vi "Check_Motility_after_Gap_Closing-2.vi"(0 "(X,Y) IN":dbl[][](array[numeric]), 1 "dR min":dbl, 5 "??? Gap closed potentially ???":bool, 7 "X":dbl, 9 "Y":dbl, 11 "Count of \ngaps between\ndots":i32, 12 "i+j (index\nof dot before\ngap closing)":i32) -> (4 "Gap closed!!!":bool, 6 "X OUT":dbl, 8 "Y OUT":dbl, 10 "[OUT] Count \nof gapes + \nnext dot in \nsearching":i32, 14 "[OUT] current dot\n# frame (column)":i32, 15 "[OUT] current # dot\nin the frame (column)":i32)   [LabVIEW 2013]
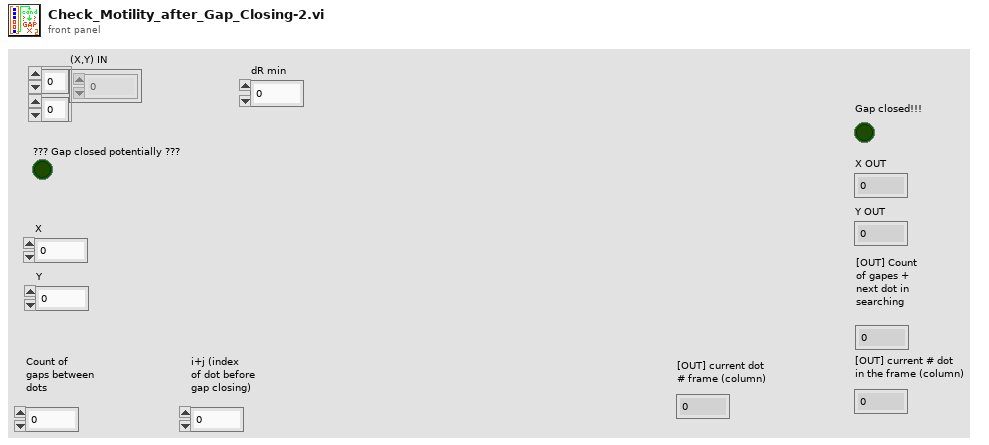
[diagram p1: front panel]
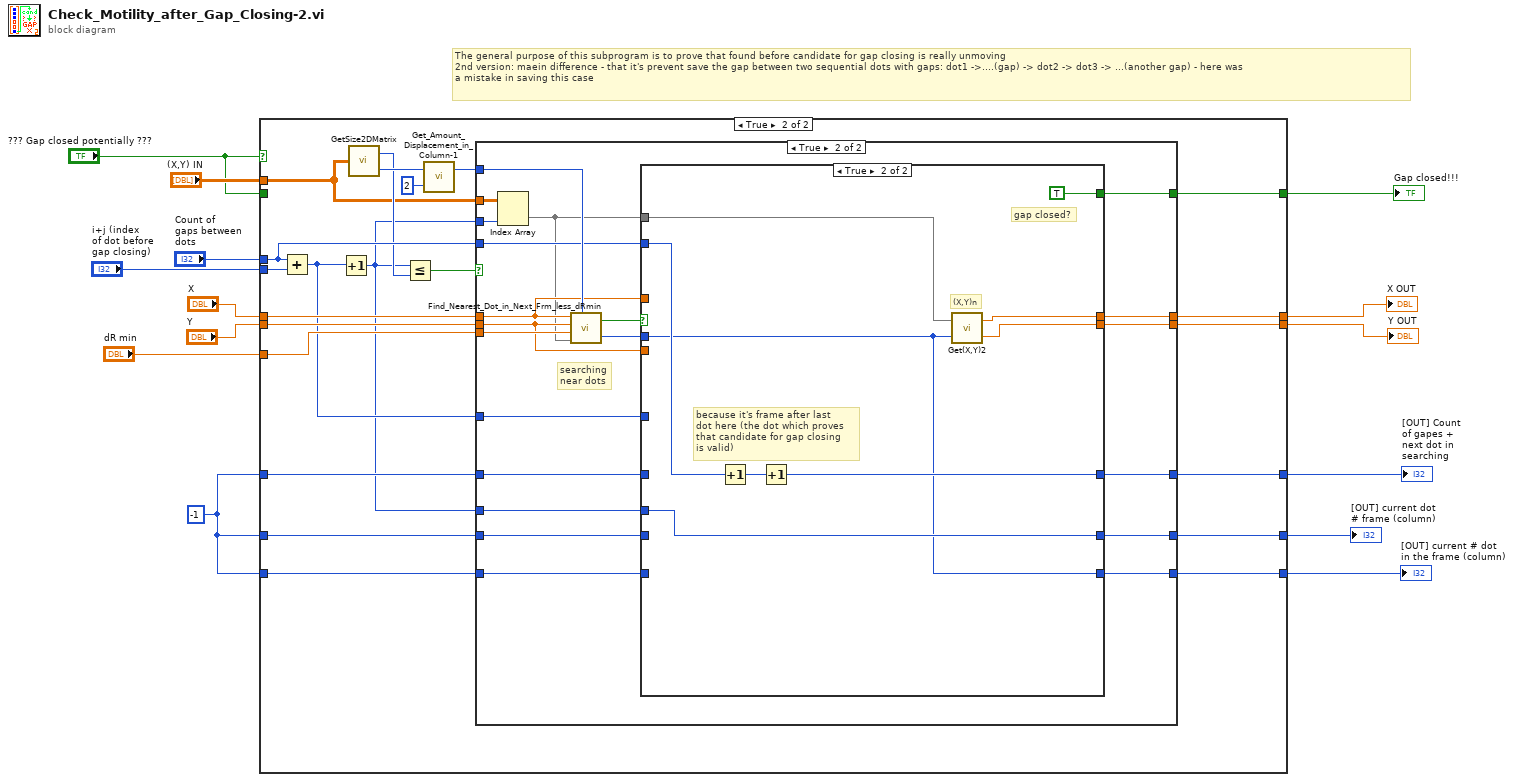
[diagram p0: block diagram]
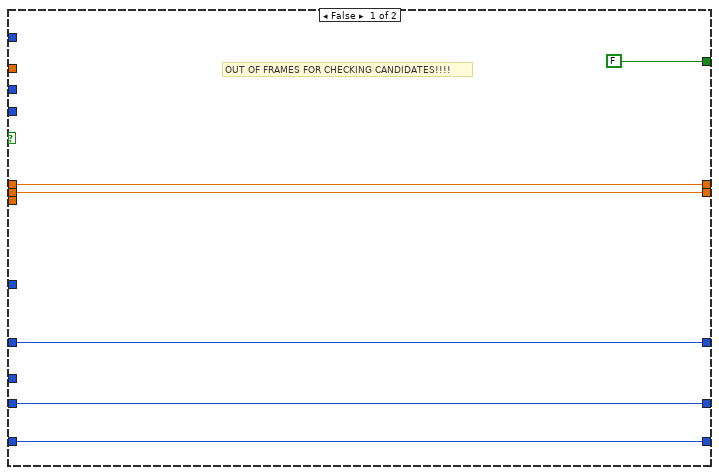
[diagram p3: hidden frame]
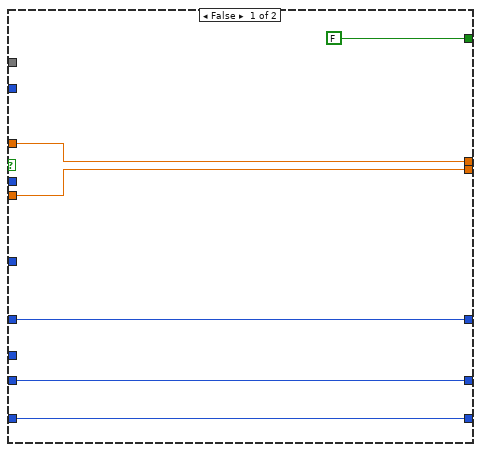
[diagram p4: hidden frame]
diagram:
  w1 = -1
  # "The general purpose of this subprogram is to prove that found before candidate for gap closing is really unmoving\n2nd version: maein difference - that it's prevent save the gap between two sequential dots with gaps: dot1 ->....(gap) -> dot2 -> dot3 -> ...(another gap) - here was\na mistake in saving this case"
  n1 = case shown="True" "??? Gap closed potentially ???" {
    tunnel: "X" -> [w20 w36]
    tunnel: "Y" -> [w19 w35]
    tunnel: "(X,Y) IN" -> [_ w22]
    tunnel: "i+j (index\nof dot before\ngap closing)" -> [_ w42]
    tunnel: "Count of \ngaps between\ndots" -> [_ w37]
    tunnel: "dR min" -> [_ w38]
    tunnel: [w20 w32] -> w8
    tunnel: [w19 w31] -> w7
    tunnel: "??? Gap closed potentially ???" -> [w18 _]
    tunnel: [w18 w33] -> w5
    tunnel: w1 -> [w17 w30]
    tunnel: [w17 w29] -> w4
    tunnel: w1 -> [w16 w28]
    tunnel: w1 -> [w15 w27]
    tunnel: [w16 w26] -> w3
    tunnel: [w15 w25] -> w2
    frame False {
    }
    frame True {
      n2 = Add(x=w37, y=w42) -> (x+y=w34:i32)
      n3 = Increment(x=w34) -> (x+1=w21:i32)
      n4 = call "GetSize2DMatrix.vi"("Array IN (2D)"=w22) -> ("# Cols"=w23:i32, "# Rows"=w41:i32)
      n5 = Less Or Equal?(x=w21, y=w23) -> (x <= y?=w24:bool)
      n6 = call "Get_Amount_Displacement_in_Column-1.vi"("multiplier"=2 ("y"), "# Rows"=w41) -> ("Displ amount"=w39:i32)  [unwired: 1 out]
      n7 = case shown="True" w24 {
        tunnel: w39 -> [_ w69]
        tunnel: w38 -> [_ w68]
        tunnel: w37 -> [_ w65]
        tunnel: w36 -> [w47 w64]
        tunnel: w35 -> [w46 w63]
        tunnel: w34 -> [_ w62]
        tunnel: [FALSE w61] -> w33
        tunnel: [w47 w60] -> w32
        tunnel: [w46 w59] -> w31
        tunnel: w30 -> [w45 w58]
        tunnel: [w45 w57] -> w29
        tunnel: w28 -> [w44 w56]
        tunnel: w27 -> [w43 w55]
        tunnel: [w44 w54] -> w26
        tunnel: [w43 w53] -> w25
        tunnel: w21 -> [_ w52]
        tunnel: w22 -> [_ w51]
        tunnel: w21 -> [_ w50]
        frame False {
          # "OUT OF FRAMES FOR CHECKING CANDIDATES!!!!"
        }
        frame True {
          # "searching\nnear dots"
          n8 = Index Array(array=w51, index (col)=w50) -> (element=w49:dbl[])  [unwired: 1 in]
          n9 = call "Find_Nearest_Dot_in_Next_Frm_less_dRmin.vi"("X"=w64, "Y"=w63, "dR min"=w68, "n+1 frame\ncolumn (X,Y)"=w49, "Max number\nof dots in \ncolumn (X,Y)"=w69) -> ("Any dots found?"=w67:bool, "index of the dot \nwith minimal displ"=w66:i32)
          n10 = case shown="True" w67 {
            tunnel: w66 -> [_ w76]
            tunnel: w65 -> [_ w80]
            tunnel: w64 -> [w74 _]
            tunnel: w63 -> [w73 _]
            tunnel: w62 -> [_ _]
            tunnel: w49 -> [_ w84]
            tunnel: [FALSE TRUE] -> w61
            tunnel: [w74 w83] -> w60
            tunnel: [w73 w81] -> w59
            tunnel: w58 -> [w72 _]
            tunnel: [w72 w78] -> w57
            tunnel: w56 -> [w71 _]
            tunnel: w55 -> [w70 _]
            tunnel: [w71 w77] -> w54
            tunnel: [w70 w76] -> w53
            tunnel: w52 -> [_ w77]
            frame False {
            }
            frame True {
              # "gap closed?"
              # "because it's frame after last \ndot here (the dot which proves \nthat candidate for gap closing\nis valid)"
              # "(X,Y)n"
              n11 = Increment(x=w80) -> (x+1=w79:i32)
              n12 = Increment(x=w79) -> (x+1=w78:i32)
              n13 = call "Get(X,Y)2.vi"("[IN] index of (X,Y)"=w76, "[IN] Array coordi\nnates (X,Y) in Frame"=w84) -> ("[OUT] Y"=w81:dbl, "[OUT] X"=w83:dbl)
            }
          }
        }
      }
    }
  }
  "X OUT" <- w8
  "Y OUT" <- w7
  "Gap closed!!!" <- w5
  "[OUT] Count \nof gapes + \nnext dot in \nsearching" <- w4
  "[OUT] current dot\n# frame (column)" <- w3
  "[OUT] current # dot\nin the frame (column)" <- w2
